vi "Stop Core Wrapper.vi"(10 "final error code":i32, 11 "Instr in":refnum<class "Instr Actor.lvclass">) -> (0 "error out":errorcluster, 3 "Instr out":refnum<class "Instr Actor.lvclass">)   [LabVIEW 2014, in "Instrument Library.lvlib" / "Instr Actor.lvclass"]
uses:
  Instr Actor.lvclass
  Instr Actor.lvclass/Instr Actor.ctl
  reusable/Instrument/Instrument.lvclass/Instrument.ctl
  SuperActor/Ex Nested.lvclass/Ex Nested.ctl
  SuperActor/Read Log Session.vi
  reusable/Instrument/Read name.vi
  <userlib>/_Session Fwk/Session - Root.lvclass
  reusable/Session APIs/Session Log/System Log.lvclass
  reusable/Instrument/Instrument.lvclass
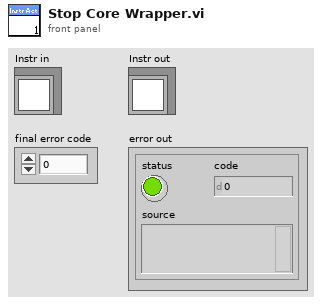
[diagram p1: front panel]
types:
  T1 = typedef "Session - Root.lvclass/Session Handle.ctl" = refnum<data-value>
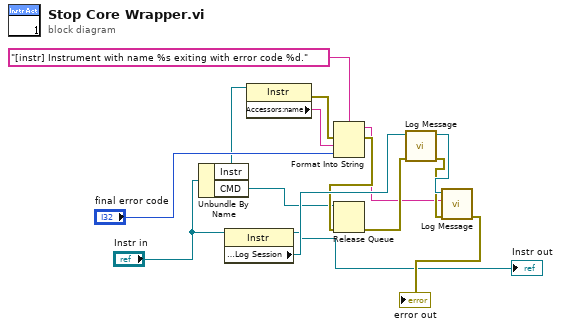
[diagram p0: block diagram]
diagram:
  n1 = Unbundle By Name("Instr in") -> ("Instr"=w2:refnum<class "Instrument.lvclass">, "CMD"=w1:refnum<queue>)
  n2 = property class="Instr"(reference="Instr in") -> (reference out=→"Instr out":refnum<class "Instr Actor.lvclass">, "Accessors:Log Session"=w10:T1)  [unwired: 1 in, 1 out]
  n3 = property class="Instr"(reference=w2) -> (error out=w8:errorcluster, "Accessors:name"=w4:string)  [unwired: 1 in, 1 out]
  n4 = Format Into String(format string="[instr] Instrument with name %s exiting with error code %d.", error in=w8, w4, "final error code") -> (resulting string=w5:string, error out=w9:errorcluster)  [unwired: 1 in]
  n5 = Release Queue(queue=w1, error in (no error)=w9) -> (error out=w11:errorcluster)  [unwired: 1 in, 2 out]
  n6 = call "Log Message.vi"("error in"=w11, "session in"=w10) -> ("error out"=w12:errorcluster, "session out"=w13:T1)  [unwired: 8 in]
  n7 = call "Log Message.vi"("error in"=w12, "MSG In"=w5, "session in"=w13) -> ("error out"=→"error out":errorcluster)  [unwired: 7 in, 1 out]
